vi "MccHat_query.vi"(7 "command":string, 8 "error in":errorcluster, 11 "conn_id_in":refnum<k5>) -> (0 "error out":errorcluster, 2 "string_array":string[](array[string]), 3 "conn_id_out":refnum<k5>, 4 "status":bool, 5 "string_raw":string)   [LabVIEW 2019]
panel:
  out "i":i32
  out "string_rest":string
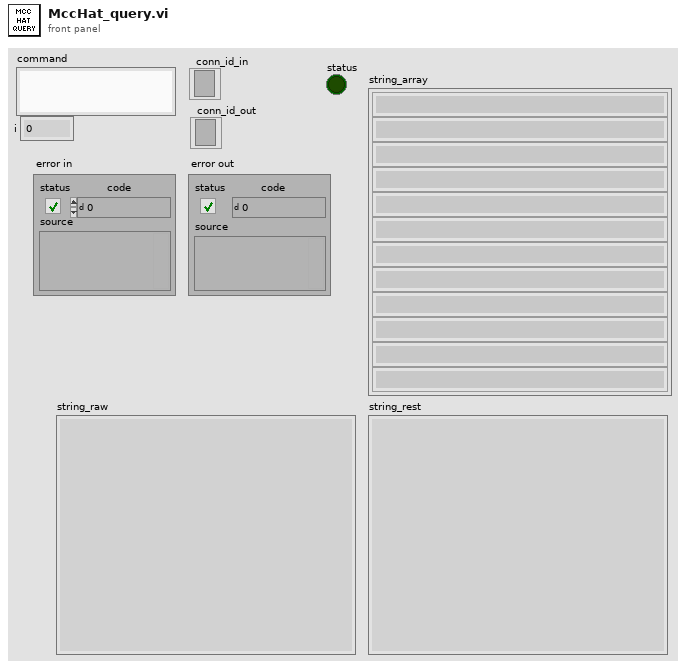
[diagram p1: front panel]
types:
  T1 = enum16{"Standard", "Buffered", "CRLF", "Immediate"}
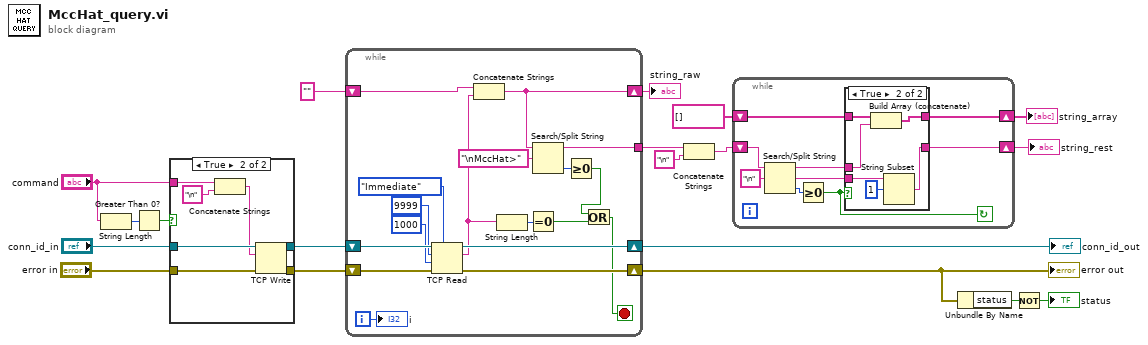
[diagram p0: block diagram]
diagram:
  n1 = String Length(string="command") -> (length=w8:i32)
  n2 = Greater Than 0?(x=w8) -> (x > 0?=w7:bool)
  n3 = case shown="True" w7 {
    tunnel: "error in" -> [w20 w28]
    tunnel: [w20 w27] -> w18
    tunnel: [w21 w26] -> w17
    tunnel: "conn_id_in" -> [w21 w25]
    tunnel: "command" -> [_ w22]
    frame False {
    }
    frame True {
      n4 = Concatenate Strings(w22, "\n" ("string")) -> (w24:string)
      n5 = TCP Write(connection ID=w25, data in=w24, error in (no error)=w28) -> (connection ID out=w26:refnum<k5>, error out=w27:errorcluster)  [unwired: 1 in, 1 out]
    }
  }
  n6 = while {
    shift-right: [w41] -> w14
    shift-left: w18 -> [w46]
    shift-right: [w42] -> w16
    shift-left: w17 -> [w45]
    shift-right: [w35] -> w10
    shift-left: "" ("string") -> [w40]
    tunnel: [w34] -> w2
    i -> [w38]
    stop <- w31 stop-if-true
    n7 = TCP Read(connection ID=w45, bytes to read=9999, error in (no error)=w46, 7:T1."Immediate" ("mode (standard)"), 9:1000 ("timeout ms (25000)")) -> (connection ID out=w42:refnum<k5>, data out=w33:string, error out=w41:errorcluster)
    n8 = Concatenate Strings(w40, w33) -> (w35:string)
    n9 = String Length(string=w33) -> (length=w32:i32)
    n10 = Equal To 0?(x=w32) -> (x = 0?=w29:bool)
    n11 = Search/Split String(string=w35, search string/char (-)="\nMccHat>") -> (substring before match=w34:string, offset of match=w36:i32)  [unwired: 1 in, 1 out]
    n12 = Greater Or Equal To 0?(x=w36) -> (x >= 0?=w30:bool)
    n13 = Or(x=w30, y=w29) -> (x .or. y?=w31:bool)
    "i" <- w38
  }
  "error out" <- w14
  "string_raw" <- w10
  "conn_id_out" <- w16
  n14 = Concatenate Strings(w2, "\n" ("search string/char (-)")) -> (w3:string)
  n15 = while {
    shift-right: [w51] -> w4
    shift-left: w3 -> [w49]
    shift-right: [w47] -> w6
    shift-left: string[] [] ("string") -> [w48]
    stop <- w50 continue-if-true
    n16 = Search/Split String(string=w49, search string/char (-)="\n") -> (substring before match=w52:string, match + rest of string=w53:string, offset of match=w54:i32)  [unwired: 1 in]
    n17 = Greater Or Equal To 0?(x=w54) -> (x >= 0?=w50:bool)
    n18 = case shown="True" w50 {
      tunnel: w53 -> [_ w63]
      tunnel: w52 -> [w56 w58]
      tunnel: [w56 w61] -> w51
      tunnel: w48 -> [w57 w60]
      tunnel: [w57 w59] -> w47
      frame False {
      }
      frame True {
        n19 = Build Array (concatenate)(w60, w58) -> (w59:string[])
        n20 = String Subset(string=w63, offset (0)=1) -> (substring=w61:string)  [unwired: 1 in]
      }
    }
  }
  "string_array" <- w6
  "string_rest" <- w4
  n21 = Unbundle By Name(w14) -> ("status"=w13:bool)
  n22 = Not(x=w13) -> (.not. x?=→"status":bool)
